vi "AlliGator Draw Tick Labels.vi"(4 "Label Distance (tick unit)":dbl=2.0, 5 "Font, Size & Style":T4, 6 "Text Color":u32, 7 "Overlay Group":string, 8 "error in (no error)":errorcluster, 9 "Phasor Plot Reference Points":T5, 10 "Tick Label Data":T1[](array[typedef]), 11 "Refnum in":T3) -> (0 "error out":errorcluster, 3 "Refnum out":T3)   [LabVIEW 2021, in "AlliGator Phasor Plot.lvlib"]
doc: "Draws UC or SEPL tick labels in the Phasor Plot image."
uses:
  AlliGator Phasor Plot.lvlib
  Phasor Ratio/AlliGator Phasor Plot Reference Points.ctl
  <vilib>/vision/Image Controls.llb/IMAQ Image.ctl
  Phasor/Phasor SEPL Tick Data.ctl
  Phasor/Phasor (g, s).ctl
  Strings/Strings.lvlib
  Phasor Ratio/AlliGator Phasor Ratio.lvlib
  Phasor/Phasor.lvlib
panel:
  # "see the AlliGator License on the block diagram (Ctrl+E or Window:Show Block Diagram)"
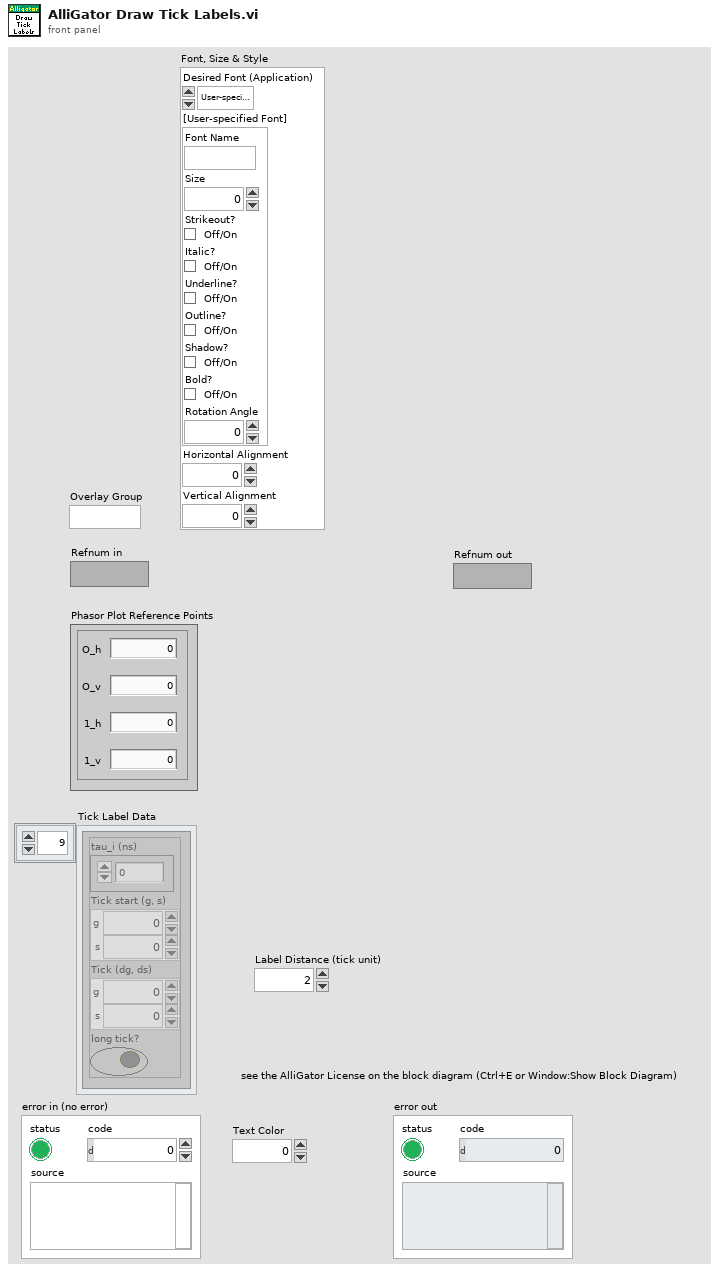
[diagram p1: front panel]
types:
  T1 = typedef "Phasor.lvlib/Phasor SEPL Tick Data.ctl" = cluster{"tau_i (ns)":dbl, "Tick start (g, s)":T2, "Tick (dg, ds)":T2, "long tick?":bool}
  T2 = typedef "Phasor.lvlib/Phasor (g, s).ctl" = cluster{"g":dbl, "s":dbl}
  T3 = typedef "IMAQ Image.ctl" = refnum<image>
  T4 = cluster{"Desired Font (Application)":enum16{"User-specified Font", "Application Font", "System Font", "Dialog Font"}, "[User-specified Font]":cluster{"Font Name":string, "Size":i16, "Strikeout?":bool, "Italic?":bool, "Underline?":bool, "Outline?":bool, "Shadow?":bool, "Bold?":bool, "Rotation Angle":dbl}, "Horizontal Alignment":i16, "Vertical Alignment":i16}
  T5 = typedef "AlliGator Phasor Ratio.lvlib/AlliGator Phasor Plot Reference Points.ctl" = cluster{"O_h":dbl, "O_v":dbl, "1_h":dbl, "1_v":dbl}
  T6 = cluster{"Phasor Plot x":dbl, "Phasor Plot y":dbl}
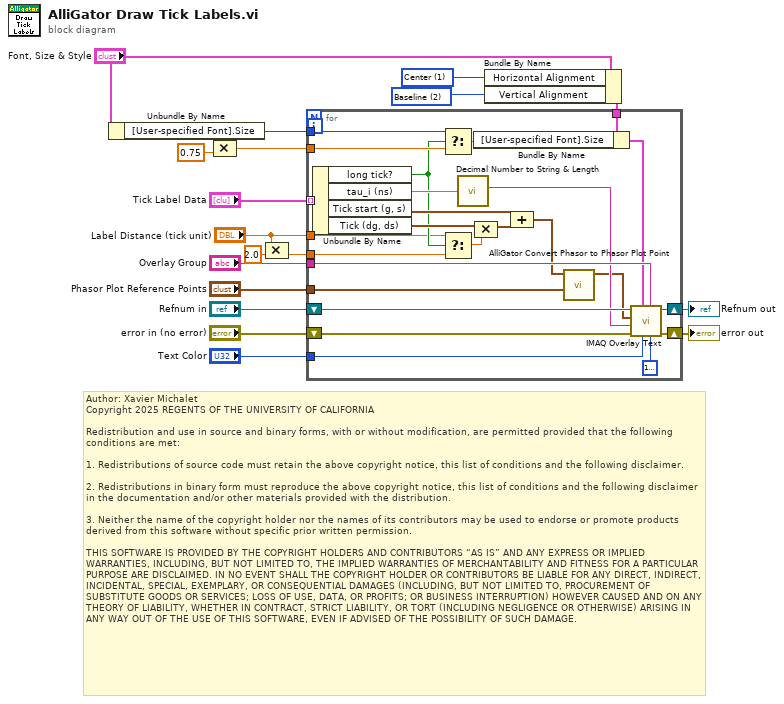
[diagram p0: block diagram]
diagram:
  w8 = i16 2 items=["Bottom", "Top", "Baseline"] ("Vertical Alignment")
  w9 = i16 1 items=["Left", "Center", "Right"] ("Horizontal Alignment")
  # "Author: Xavier Michalet\nCopyright 2025 REGENTS OF THE UNIVERSITY OF CALIFORNIA\n\nRedistribution and use in source and binary forms, with or without modification, are permitted provided that the following conditions are met:\n\n1. Redistributions of source code must retain the above copyright notice, this list of conditions and the following disclaimer.\n\n2. Redistributions in binary form must reproduce the above copyright notice, this list of conditions and the following disclaimer in the documentation and/or other materials provided with the distribution.\n\n3. Neither the name of the copyright holder nor the names of its contributors may be used to endorse or promote products derived from this software without specific prior written permission.\n\nTHIS SOFTWARE IS PROVIDED BY THE COPYRIGHT HOLDERS AND CONTRIBUTORS “AS IS” AND ANY EXPRESS OR IMPLIED WARRANTIES, INCLUDING, BUT NOT LIMITED TO, THE IMPLIED WARRANTIES OF MERCHANTABILITY AND FITNESS FOR A PARTICULAR PURPOSE ARE DISCLAIMED. IN NO EVENT SHALL THE COPYRIGHT HOLDER OR CONTRIBUTORS BE LIABLE FOR ANY DIRECT, INDIRECT, INCIDENTAL, SPECIAL, EXEMPLARY, OR CONSEQUENTIAL DAMAGES (INCLUDING, BUT NOT LIMITED TO, PROCUREMENT OF SUBSTITUTE GOODS OR SERVICES; LOSS OF USE, DATA, OR PROFITS; OR BUSINESS INTERRUPTION) HOWEVER CAUSED AND ON ANY THEORY OF LIABILITY, WHETHER IN CONTRACT, STRICT LIABILITY, OR TORT (INCLUDING NEGLIGENCE OR OTHERWISE) ARISING IN ANY WAY OUT OF THE USE OF THIS SOFTWARE, EVEN IF ADVISED OF THE POSSIBILITY OF SUCH DAMAGE."
  n1 = Unbundle By Name("Font, Size & Style") -> ("[User-specified Font].Size"=w6:i16)
  n2 = Compound Arithmetic op=MULTIPLY(w6, 0.75 ("value")) -> (w4:dbl)
  n3 = Compound Arithmetic op=MULTIPLY("Label Distance (tick unit)", 2.0 ("s? t:f")) -> (w2:dbl)
  n4 = Bundle By Name(cluster="Font, Size & Style", "Horizontal Alignment"=w9, "Vertical Alignment"=w8) -> (w10:T4)
  n5 = for {
    shift-right: [w38] -> w13
    shift-left: "Refnum in" -> [w39]
    shift-right: [w42] -> w15
    shift-left: "error in (no error)" -> [w43]
    tunnel: "Tick Label Data" -> [w36] mode=indexing
    tunnel: "Text Color" -> [w41]
    tunnel: "Overlay Group" -> [w40]
    tunnel: w10 -> [w37]
    tunnel: "Phasor Plot Reference Points" -> [w32]
    tunnel: w6 -> [w24]
    tunnel: w4 -> [w23]
    tunnel: "Label Distance (tick unit)" -> [w20]
    tunnel: w2 -> [w19]
    n6 = Unbundle By Name(w36) -> ("long tick?"=w21:bool, "tau_i (ns)"=w29:dbl, "Tick start (g, s)"=w35:T2, "Tick (dg, ds)"=w34:T2)
    n7 = Select(t=w24, s=w21, f=w23) -> (s? t:f=w25:dbl)
    n8 = Select(t=w20, s=w21, f=w19) -> (s? t:f=w22:dbl)
    n9 = call "Decimal Number to String & Length.vi"("Decimal Number"=w29) -> ("String"=w28:string)  [unwired: 6 in, 1 out]
    n10 = Bundle By Name(cluster=w37, "[User-specified Font].Size"=w25) -> (w26:T4)
    n11 = Compound Arithmetic op=MULTIPLY(w34, w22) -> (w33:T2)
    n12 = Compound Arithmetic op=ADD(w35, w33) -> (w31:T2)
    n13 = call "AlliGator Convert Phasor to Phasor Plot Point.vi"("Phasor Plot Reference Points"=w32, "Phasor"=w31) -> ("Phasor Plot Point"=w27:T6)  [unwired: 9 in]
    n14 = call "IMAQ Overlay Text"("BG Color (Transparent)"=u32 16777216, "Group"=w40, "Text Color (black)"=w41, "Font, Size & Style"=w26, "error in (no error)"=w43, "String"=w28, "Origin"=w27, "Image"=w39) -> ("error out"=w42:errorcluster, "Image Out"=w38:T3)  [unwired: 2 in]
  }
  "error out" <- w15
  "Refnum out" <- w13
